vi "ToDatagram.vi"(8 "error in (no error)":errorcluster, 10 "messageID":u16, 11 "ConnectMqttMsg in":refnum<class "ConnectMqttMsg.lvclass">) -> (0 "error out":errorcluster, 2 "Datagram":u8[](array[numeric]), 3 "ConnectMqttMsg out":refnum<class "ConnectMqttMsg.lvclass">)   [LabVIEW 2020, in "ConnectMqttMsg.lvclass"]
uses:
  ConnectMqttMsg.lvclass
  mqttTypedef/QosLevel.ctl
  mqttTypedef/MessageType.ctl
  ConnectMqttMsg.lvclass/ConnectMqttMsg.ctl
  BaseMqttMsg.lvclass
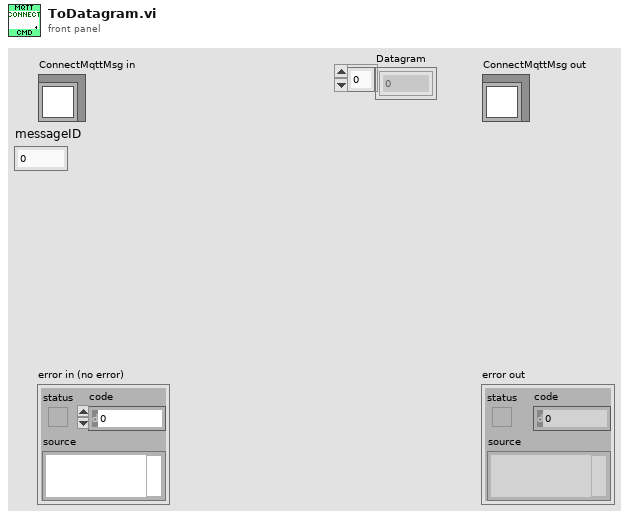
[diagram p1: front panel]
types:
  T1 = typedef "BaseMqttMsg.lvclass/MessageType.ctl" = enum32{"Reserved", "CONNECT", "CONNACK", "PUBLISH", "PUBACK", "PUBREC", "PUBREL", "PUBCOMP", "SUBSCRIBE", "SUBACK", "UNSUBSCRIBE", "UNSUBACK", "PINGREQ", "PINGRESP", "DISCONNECT", "Reserved2"}
  T2 = typedef "BaseMqttMsg.lvclass/QosLevel.ctl" = enum8{"At most once", "At least once", "Exactly once", "Reserved"}
  T3 = typedef "MQTT Client.lvclass/ConnectionFlags.ctl" = cluster{"user name":bool, "password":bool, "will retain":bool, "will flag":bool, "clean session":bool, "reserved":bool, "willQOS":T2}
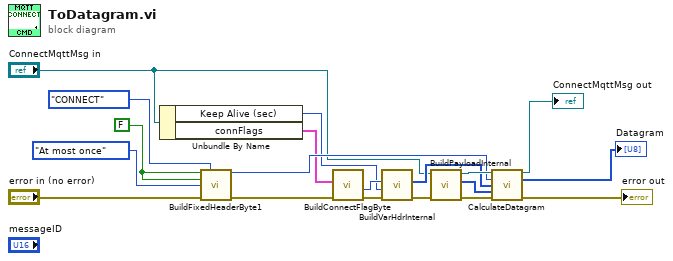
[diagram p0: block diagram]
diagram:
  w17 = FALSE
  n1 = Unbundle By Name("ConnectMqttMsg in") -> ("Keep Alive (sec)"=w2:u16, "connFlags"=w3:T3)
  n2 = call "BuildFixedHeaderByte1.vi"("retain(F)"=w17, "MessageType"=MessageType."CONNECT", "duplicate(F)"=w17, "QoS (At most once)"=QosLevel."At most once", "error in (no error)"="error in (no error)") -> ("byte1"=w11:u8, "error out"=w15:errorcluster)  [unwired: 9 in]
  n3 = call "BuildConnectFlagByte.vi"("error in (no error)"=w15, "connFlags"=w3) -> ("error out"=w14:errorcluster, "connFlagByte out"=w13:u8)  [unwired: 8 in]
  n4 = call "BuildVarHdrInternal.vi"("error in (no error)"=w14, "keepAlive(sec)"=w2, "connFlagByte"=w13) -> ("error out"=w19:errorcluster, "varHeader"=w10:u8[])  [unwired: 7 in]
  n5 = call "BuildPayloadInternal.vi"("error in (no error)"=w19, "mqttCmdConnect in"="ConnectMqttMsg in") -> ("error out"=w8:errorcluster, "payload"=w9:u8[], "mqttCmdConnect out"=w12:refnum<class "ConnectMqttMsg.lvclass">)  [unwired: 7 in]
  n6 = call-dynamic "CalculateDatagram.vi"("mqttCmd in"=w12, "FixedHeaderByte1"=w11, "variableHeader"=w10, "payload"=w9, "error in (no error)"=w8) -> ("mqttCmd out"=→"ConnectMqttMsg out":refnum<class "ConnectMqttMsg.lvclass">, "Datagram"=→"Datagram":u8[], "error out"=→"error out":errorcluster)  [unwired: 8 in]
